vi "RobotState.vi"() -> ()   [LabVIEW 2019]
uses:
  Implements/Shooter/TypeDefs/Hood_Homing_State.ctl
  Implements/Control_Panel/TypeDefs/ControlPanelColor.ctl
panel:
  out "ControlPanelRotations":dbl
  out "ControlPanelHue":dbl
  out "HoodSetpoint(deg)":dbl
  out "TurretSetpoint(deg)":dbl
  out "ShooterSetpoint(rpm)":dbl
  out "ShooterVelocity(rpm)":dbl
  out "RightDriveDistance":dbl
  out "LeftDriveDistance":dbl
  out "BottomBallDistance":dbl
  out "TopBallDistance":dbl
  out "RobotAngle":dbl
  out "TopBallPresent":bool
  out "BottomBallPresent":bool
  out "HoodAutoActive":bool
  out "TurretAutoActive":bool
  out "HoodAngle":dbl
  out "TurretAngle":dbl
  out "TopBallCount":u16
  out "BottomBallCount":u16
  out "ControlPanelColor":T1
  out "TurretHomingState":T2
  out "HoodHomingState":T2
  out "ShooterReady":bool
  out "Aimed":bool
  out "TargetAcquired":bool
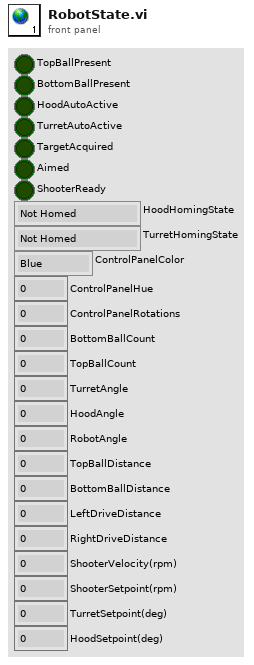
[diagram p1: front panel]
types:
  T1 = typedef "ControlPanelColor.ctl" = enum16{"Blue", "Green", "Red", "Yellow", "Unknown"}
  T2 = typedef "Hood_Homing_State.ctl" = enum16{"Not Homed", "Homing in Process", "Homing Failed", "Homing Completed"}
diagram:
